vi "Read System Metadata.vi"() -> ()   [LabVIEW 2020]
uses:
  <vilib>/httpClient/ClientHandle.ctl
  <vilib>/Skyline/Configuration/Configuration HTTP_class/NI Skyline Configuration HTTP.lvclass/NI Skyline Configuration HTTP.ctl
  <vilib>/Skyline/Configuration/Configuration HTTP_class/Open Configuration HTTP Auto.vi
  <vilib>/Skyline/Configuration/Configuration HTTP_class/Read Server URL.vi
  <vilib>/Skyline/Configuration/HTTP/Open Configuration Auto (Custom).vi
  <vilib>/Skyline/Configuration/HTTP/Configuration File Cache.vi
  <vilib>/Skyline/Configuration/HTTP/Initialize From Auto Configuration.vi
  <vilib>/httpClient/POSTBuffer.vi
  <vilib>/Skyline/Configuration/Configuration HTTP_class/NI Skyline Configuration HTTP.lvclass
  <vilib>/Skyline/Configuration/Configuration_class/NI Skyline Configuration.lvclass
  <vilib>/httpClient/LabVIEWHTTPClient.lvlib
  <vilib>/Skyline/Utilities/NI Skyline Utilities.lvlib
panel:
  out "error out":errorcluster
  out "client handle out":T1
  out "body":string
  out "Server URL":string
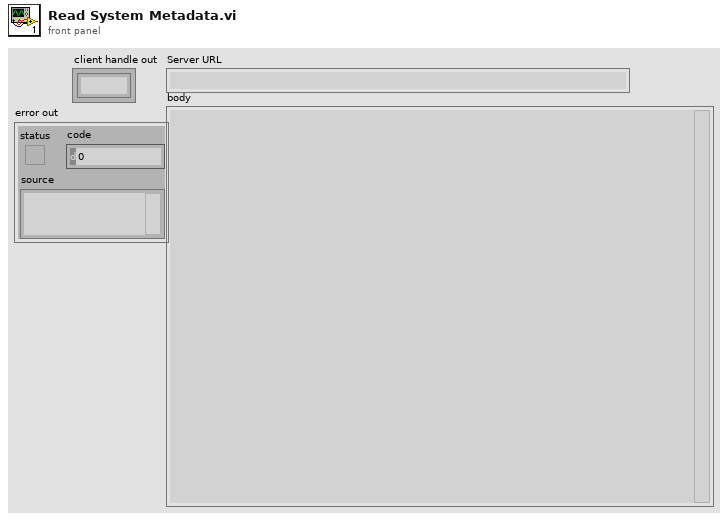
[diagram p1: front panel]
types:
  T1 = typedef "LabVIEWHTTPClient.lvlib/ClientHandle.ctl" = refnum<k1>
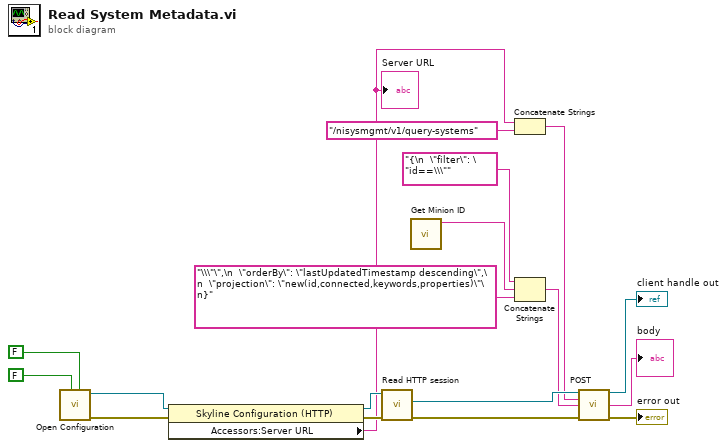
[diagram p0: block diagram]
diagram:
  n1 = call-poly <vilib>:"Open Configuration.vi"("HTTPS only?"=FALSE, "verify server?"=FALSE) -> ("error out"=w14:errorcluster, "configuration"=w15:refnum<class "NI Skyline Configuration HTTP.lvclass">)  [unwired: 8 in]
  n2 = property class="Skyline Configuration (HTTP)"(reference=w15, error in=w14) -> (reference out=w13:refnum<class "NI Skyline Configuration HTTP.lvclass">, error out=w12:errorcluster, "Accessors:Server URL"=w10:string)
  "Server URL" <- w10
  n3 = call <vilib>:"Read HTTP session.vi"("error in (no error)"=w12, "HTTP configuration in"=w13) -> ("error out"=w11:errorcluster, "http session"=w16:T1)  [unwired: 7 in, 1 out]
  n4 = call <vilib>:"Get Minion ID.vi"() -> ("minion id"=w6:string)  [unwired: 11 in]
  n5 = Concatenate Strings(w10, "/nisysmgmt/v1/query-systems" ("string")) -> (w9:string)
  n6 = Concatenate Strings("{\n  \"filter\": \"id==\\\"" ("buffer"), w6, "\\\"\",\n  \"orderBy\": \"lastUpdatedTimestamp descending\",\n  \"projection\": \"new(id,connected,keywords,properties)\"\n}" ("buffer")) -> (w4:string)
  n7 = call-poly <vilib>:"POST.vi"("client handle"=w16, "url"=w9, "buffer"=w4, "error in (no error)"=w11) -> ("client handle out"=→"client handle out":T1, "body"=→"body":string, "error out"=→"error out":errorcluster)  [unwired: 8 in, 1 out]
